vi "3. Message Helper VI and Equivalent String.vi"() -> ()   [LabVIEW 2017]
doc: "### 3. Message Helper VI and Equivalent String.vi\n\n#### Overview\n\nDemonstrates string syntax format for message communications within the CSM framework.\n\n#### Introduction\n\nThis example explains the following types of string syntax format of inter-CSM-module message communication:\n- Sync message\n- Async message with reply\n- Async message without reply\n- Broadcasting a normal status string\n- Broadcasting an interrupt or a high-priority status string\n- Registering a status\n- Unregistering a status\n\nYou can use the LabVIEW API to build these strings, or you can create these strings manually by following message rules."
uses:
  user.lib/_NEVSTOP/Communicable State Machine(CSM)/_Polymophic/Build Synchronous Message with Arguments.vi
  user.lib/_NEVSTOP/Communicable State Machine(CSM)/_Polymophic/Build Asynchronous Message with Arguments.vi
  user.lib/_NEVSTOP/Communicable State Machine(CSM)/_Polymophic/Build Interrupt Status Message.vi
  user.lib/_NEVSTOP/Communicable State Machine(CSM)/_Polymophic/Build No-Reply Asynchronous Message with Arguments.vi
  user.lib/_NEVSTOP/Communicable State Machine(CSM)/_Polymophic/Build Normal Status Message.vi
  user.lib/_NEVSTOP/Communicable State Machine(CSM)/_Polymophic/Build Unregister Status Message.vi
  user.lib/_NEVSTOP/Communicable State Machine(CSM)/_Polymophic/Build Register Status Message.vi
  user.lib/_NEVSTOP/Communicable State Machine(CSM)/Communicable State Machine.lvlib
panel:
  out "Equivalent String (Register Status)":string="Status Changed-> <all>"
  out "Equivalent String (Unregister Status)":string="Status Changed >> Argument-> <all>"
  out "Equivalent String (Async without reply Message)":string="State >> Argument->DestModuleName"
  out "Equivalent String (Interrupt Status)":string="Status Changed >> Argument-> <all>"
  out "Equivalent String (Normal Status)":string="Status Changed-> <all>"
  out "Equivalent String (Async Message)":string="State >> Argument->DestModuleName"
  out "Equivalent String (Sync Message)":string="State >> Argument@DestModuleName"
  # "#CSM-Example Overview\n\nDemonstrates string syntax format for message communications within the CSM framework."
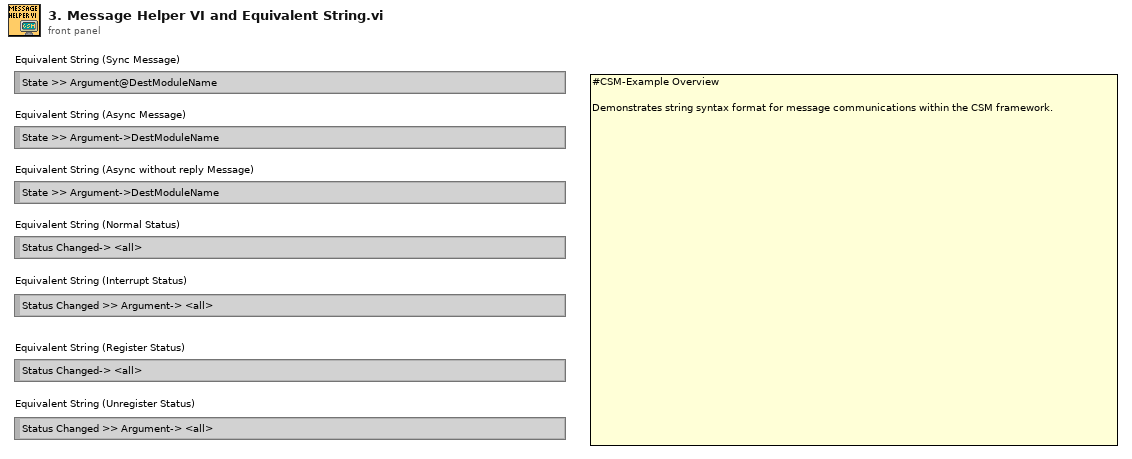
[diagram p1: front panel]
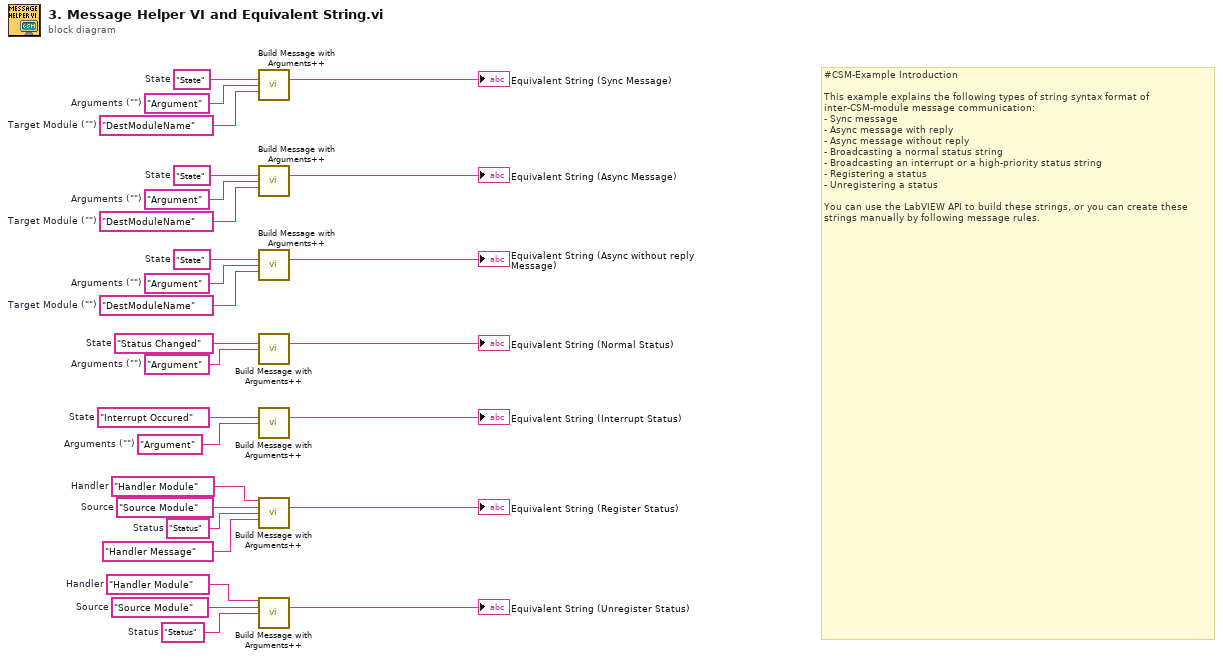
[diagram p0: block diagram]
diagram:
  w2 = "Handler Module"  # Handler
  w3 = "Handler Module"  # Handler
  w9 = "Status"  # Status
  w7 = "Status"  # Status
  w6 = "Source Module"  # Source
  w8 = "Source Module"  # Source
  w10 = "Argument"  # Arguments ("")
  w16 = "Argument"  # Arguments ("")
  w15 = "DestModuleName"  # Target Module ("")
  w17 = "State"  # State
  w12 = "Argument"  # Arguments ("")
  w13 = "Interrupt Occured"  # State
  w11 = "Status Changed"  # State
  w21 = "Argument"  # Arguments ("")
  w22 = "DestModuleName"  # Target Module ("")
  w20 = "State"  # State
  w26 = "Argument"  # Arguments ("")
  w25 = "DestModuleName"  # Target Module ("")
  w27 = "State"  # State
  # "#CSM-Example Introduction\n\nThis example explains the following types of string syntax format of inter-CSM-module message communication:\n- Sync message\n- Async message with reply\n- Async message without reply\n- Broadcasting a normal status string\n- Broadcasting an interrupt or a high-priority status string\n- Registering a status\n- Unregistering a status\n\nYou can use the LabVIEW API to build these strings, or you can create these strings manually by following message rules."
  n1 = call-poly "Build Message with Arguments++.vi"("State With Arguments"=w27, "Arguments (\"\")"=w26, "Target Module (\"\")"=w25) -> ("CSM Message String"=→"Equivalent String (Sync Message)":string)  [unwired: 12 in]
  n2 = call-poly "Build Message with Arguments++.vi"("State With Arguments"=w20, "Arguments (\"\")"=w21, "Target Module (\"\")"=w22) -> ("CSM Message String"=→"Equivalent String (Async Message)":string)  [unwired: 12 in]
  n3 = call-poly "Build Message with Arguments++.vi"("State With Arguments"=w17, "Arguments (\"\")"=w16, "Target Module (\"\")"=w15) -> ("CSM Message String"=→"Equivalent String (Async without reply Message)":string)  [unwired: 12 in]
  n4 = call-poly "Build Message with Arguments++.vi"("State With Arguments"=w11, "Arguments (\"\")"=w10) -> ("CSM Message String"=→"Equivalent String (Normal Status)":string)  [unwired: 13 in]
  n5 = call-poly "Build Message with Arguments++.vi"("State With Arguments"=w13, "Arguments (\"\")"=w12) -> ("CSM Message String"=→"Equivalent String (Interrupt Status)":string)  [unwired: 13 in]
  n6 = call-poly "Build Message with Arguments++.vi"("Target CSM"=w2, "Source CSM (* as Default)"=w8, "Status"=w9, "API (If \"\", Same As \"Status\")"="Handler Message" ("Response Message (if \"\", same as Source Message)")) -> ("CSM Message String"=→"Equivalent String (Register Status)":string)  [unwired: 11 in]
  n7 = call-poly "Build Message with Arguments++.vi"("Target CSM"=w3, "Source CSM (* as Default)"=w6, "Status"=w7) -> ("CSM Message String"=→"Equivalent String (Unregister Status)":string)  [unwired: 12 in]
